vi "RP Log Error.vi"(8 "error in":errorcluster, 11 "Log File Path":path=path "C:/Data/RP Log.txt") -> ()   [LabVIEW 2024]
uses:
  <vilib>/Utility/error.llb/DialogType.ctl
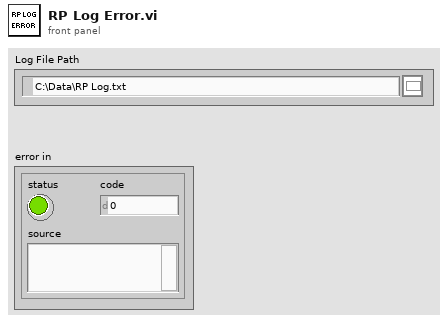
[diagram p1: front panel]
types:
  T1 = enum16{"open", "replace", "create", "open or create", "replace or create", "replace or create with confirmation"}
  T2 = typedef "DialogType.ctl" = u16
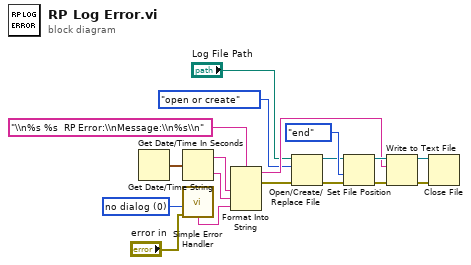
[diagram p0: block diagram]
diagram:
  w18 = T2 0 items=["no dialog", "OK message", "continue or stop message", "OK message + warnings", "continue/stop + warnings"] ("type of dialog (OK msg:1)")
  n1 = Get Date/Time In Seconds() -> (seconds since 1Jan1904=w8:timestamp)
  n2 = Get Date/Time String(seconds (now)=w8) -> (date string=w7:string, time string=w6:string)  [unwired: 2 in]
  n3 = call <vilib>:"Simple Error Handler.vi"("type of dialog (OK msg:1)"=w18, "error in (no error)"="error in") -> ("message"=w4:string)  [unwired: 3 in, 4 out]
  n4 = Format Into String(format string="\\n%s %s  RP Error:\\nMessage:\\n%s\\n", w7, w6, w4) -> (resulting string=w3:string, error out=w9:errorcluster)  [unwired: 2 in]
  n5 = Open/Create/Replace File(file path (use dialog)="Log File Path", error in=w9, operation (0:open)=T1."open or create") -> (refnum out=w10:refnum<file>, error out=w13:errorcluster)  [unwired: 3 in, 1 out]
  n6 = Set File Position(refnum=w10, from (0:start)=enum16{"start", "end", "current"}."end", error in=w13) -> (refnum out=w11:refnum<file>, error out=w14:errorcluster)  [unwired: 1 in]
  n7 = Write to Text File(file (use dialog)=w11, text=w3, error in=w14) -> (refnum out=w16:refnum<file>, error out=w15:errorcluster)  [unwired: 1 in, 1 out]
  n8 = Close File(refnum=w16, error in=w15) -> ()  [unwired: 2 out]
